vi "practice1-case2-Merve Polat.vi"() -> ()   [LabVIEW 2024]
panel:
  out "Numeric 4":dbl
  out "Ch1 Outflow Tube(4-2)":u32(colorbox)
  out "appended array":i8[](array[numeric]) format="%02x"
  out "Byte 2(8bit integer)":i8
  out "Byte 1(8bit integer)":i8
  out "Numeric 5":dbl
  out "Numeric 3":dbl
  out "Numeric 2":dbl
  out "Numeric":dbl
  out "element":u32
  out "Ch1 Current Digit Color(7-5)":u32(colorbox)
  out "Ch1 Voltage Digit Color(4-2)":u32(colorbox)
  out "Ch1 Frame Color(7-5)":u32(colorbox)
  out "1 o":u32[](array[numeric])
  out "2":u32[](array[numeric])
  out "color":u32[](array[colorbox])
  out "?":string
  out "?":string
  out "?":string
  out "?":string
  in  "Byte Array":u8[](array[numeric]) format="%02x"
  # "Ch1 Current Digit Color"
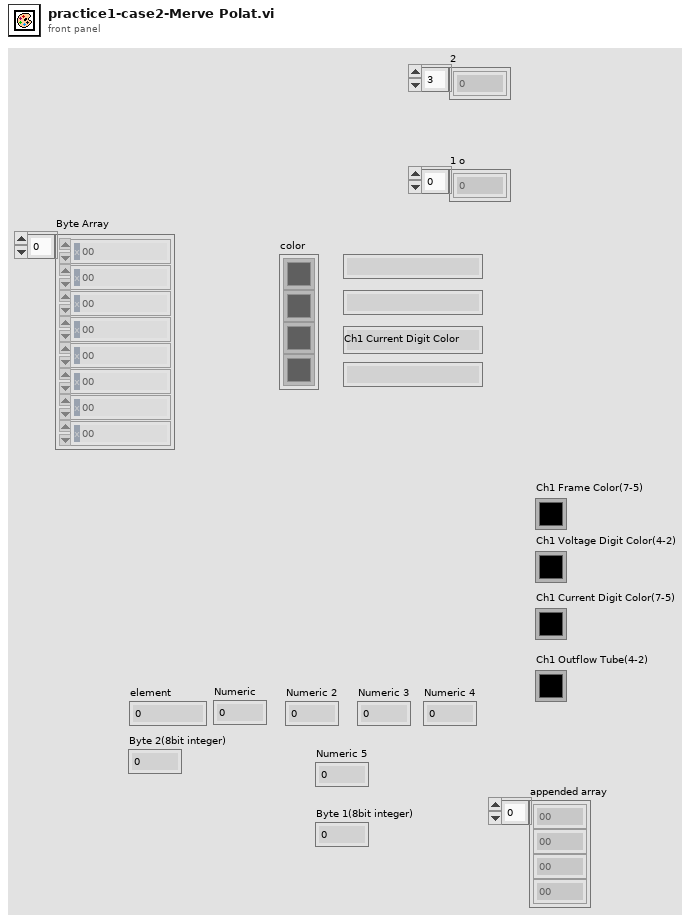
[diagram p1: front panel]
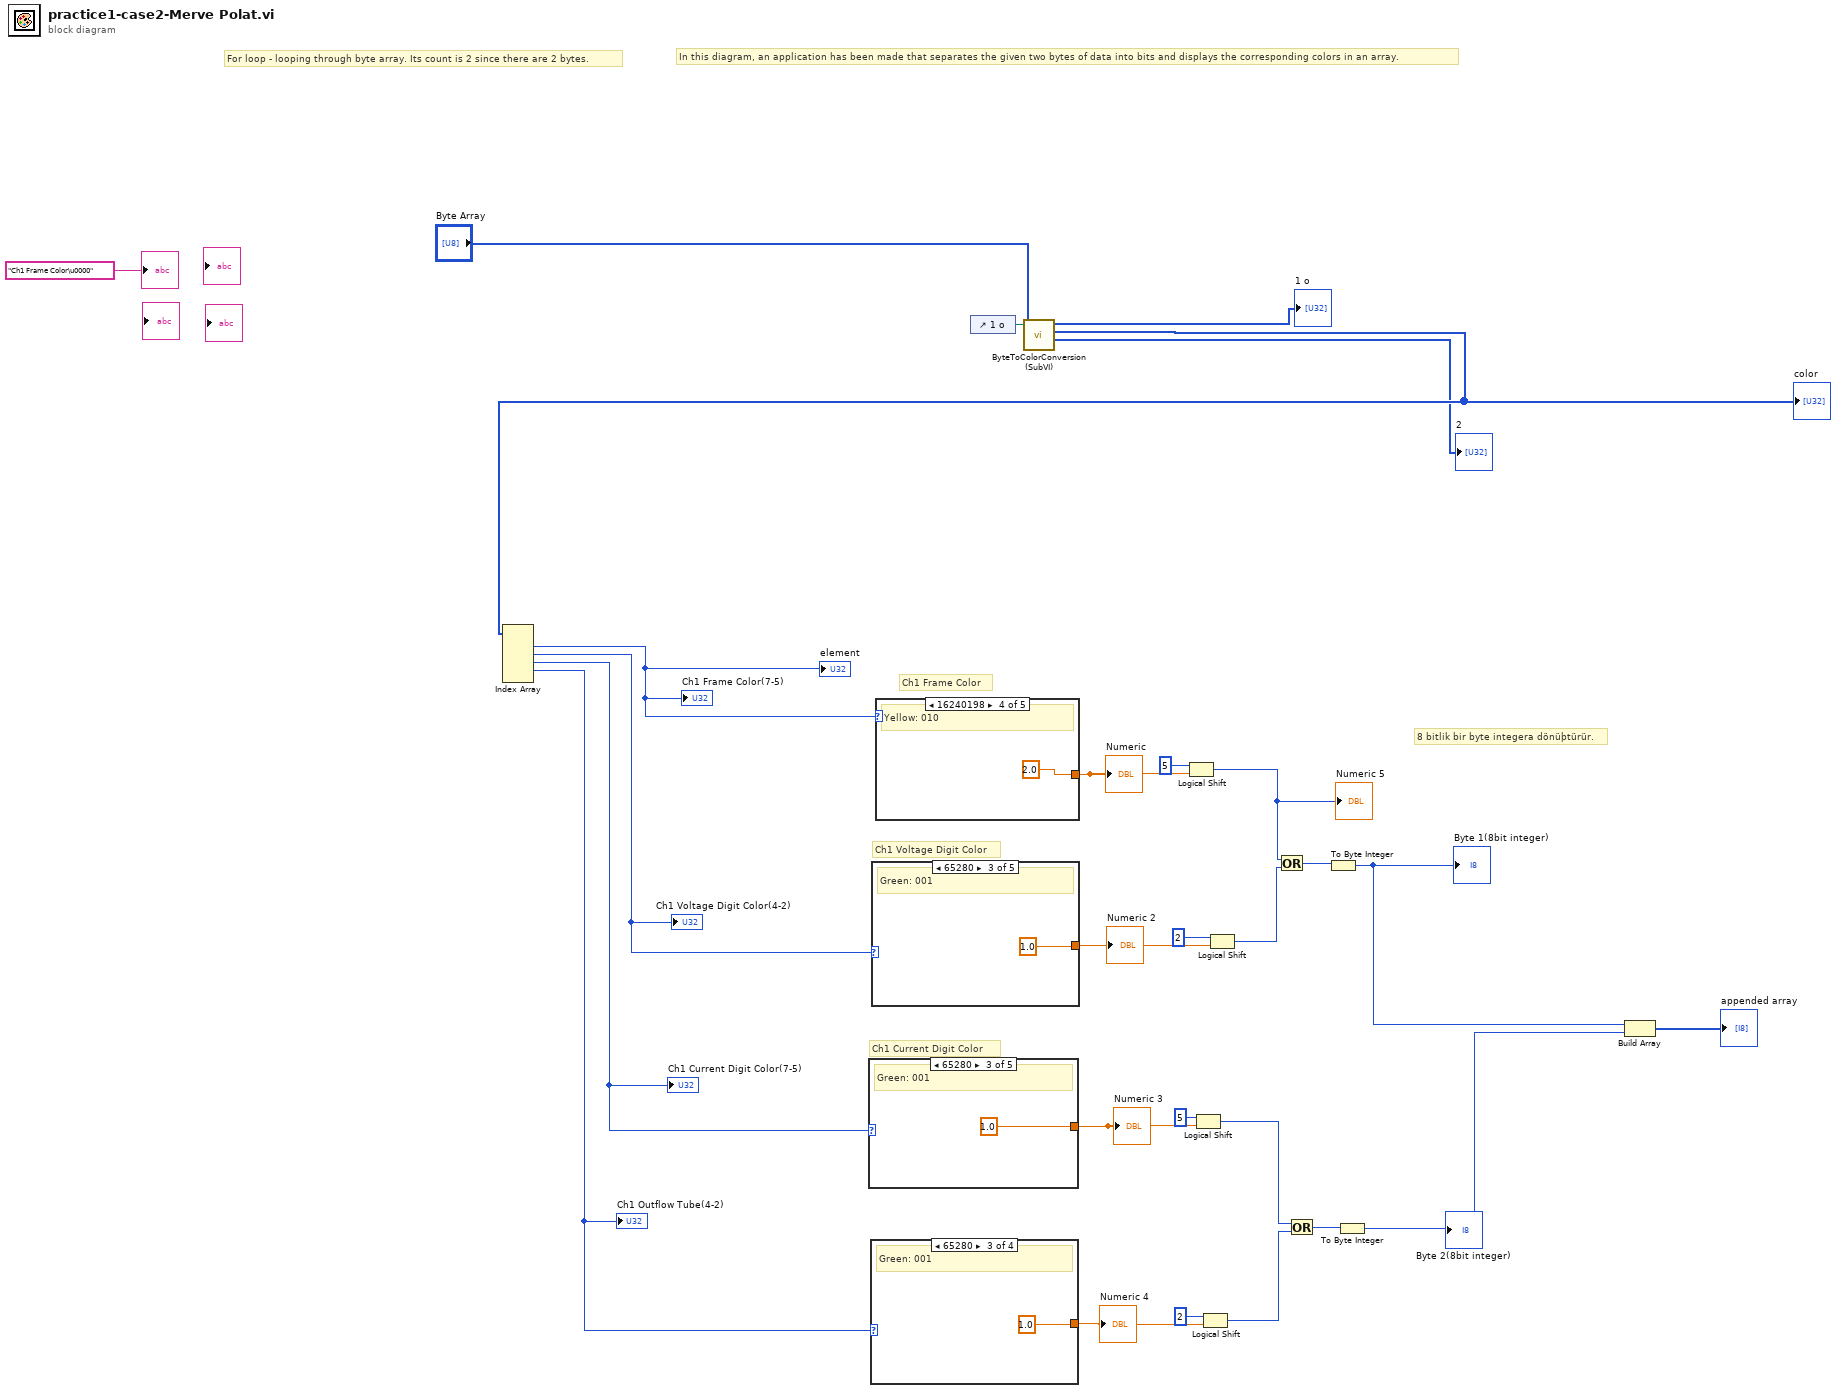
[diagram p0: block diagram]
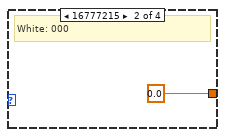
[diagram p3: hidden frame]
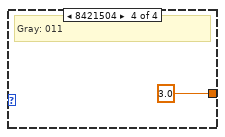
[diagram p4: hidden frame]
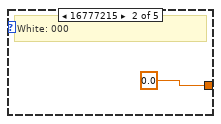
[diagram p6: hidden frame]
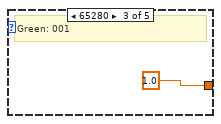
[diagram p7: hidden frame]
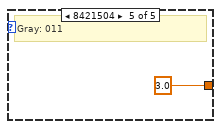
[diagram p8: hidden frame]
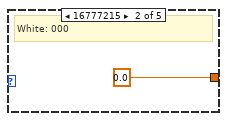
[diagram p10: hidden frame]
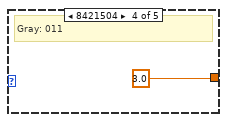
[diagram p11: hidden frame]
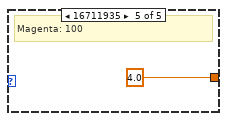
[diagram p12: hidden frame]
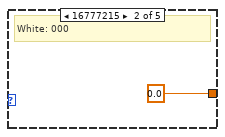
[diagram p14: hidden frame]
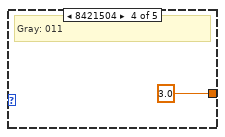
[diagram p15: hidden frame]
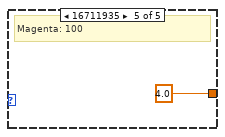
[diagram p16: hidden frame]
diagram:
  # "8 bitlik bir byte integera dönüþtürür."
  # "Ch1 Current Digit Color"
  # "Ch1 Voltage Digit Color"
  # "Ch1 Frame Color"
  # "In this diagram, an application has been made that separates the given two bytes of data into bits and displays the corresponding colors in an array."
  # "For loop - looping through byte array. Its count is 2 since there are 2 bytes."
  n1 = control-ref of="1 o"() -> (w3:refnum<vi>)
  n2 = call "ByteToColorConversion (SubVI).vi"("Byte Array"="Byte Array", "Array in"=w3) -> ("2"=→"2":u32[], "1 o 2"=w13:u32[], "1 o"=→"1 o":u32[])  [unwired: 7 in]
  "color" <- w13
  n3 = Index Array "Index Array"(array=w13) -> (element #1=w26:u32, element #2=w10:u32, element #3=w12:u32, element #4=w9:u32)  [unwired: 5 in, 1 out]
  "Ch1 Frame Color(7-5)" <- w26
  "Ch1 Voltage Digit Color(4-2)" <- w10
  "Ch1 Current Digit Color(7-5)" <- w12
  "element" <- w26
  "Ch1 Outflow Tube(4-2)" <- w9
  n4 = case shown="65280" w12 {
    tunnel: [_ 0.0 ("Numeric 3") 1.0 ("Numeric 3") 3.0 ("Numeric 3") 4.0 ("Numeric 3")] -> w19
    frame Default {
      # "None of these case is true"
    }
    frame 16777215 {
      # "White: 000"
    }
    frame 65280 {
      # "Green: 001"
    }
    frame 8421504 {
      # "Gray: 011"
    }
    frame 16711935 {
      # "Magenta: 100"
    }
  }
  "Numeric 3" <- w19
  n5 = case shown="65280" w9 {
    tunnel: [_ 0.0 ("Numeric") 1.0 ("Numeric") 3.0 ("Numeric")] -> w11
    frame Default {
      # "None of these case is true"
    }
    frame 16777215 {
      # "White: 000"
    }
    frame 65280 {
      # "Green: 001"
    }
    frame 8421504 {
      # "Gray: 011"
    }
  }
  "Numeric 4" <- w11
  n6 = case shown="65280" w10 {
    tunnel: [_ 0.0 ("Numeric") 1.0 ("Numeric") 3.0 ("Numeric") 4.0 ("Numeric")] -> w22
    frame Default {
      # "None of these case is true"
    }
    frame 16777215 {
      # "White: 000"
    }
    frame 65280 {
      # "Green: 001"
    }
    frame 8421504 {
      # "Gray: 011"
    }
    frame 16711935 {
      # "Magenta: 100"
    }
  }
  "Numeric 2" <- w22
  n7 = case shown="16240198" w26 {
    tunnel: [_ 0.0 ("Numeric") 1.0 ("Numeric") 2.0 ("Numeric") 3.0 ("Numeric")] -> w24
    frame Default {
      # "None of these case is true"
    }
    frame 16777215 {
      # "White: 000"
    }
    frame 65280 {
      # "Green: 001"
    }
    frame 16240198 {
      # "Yellow: 010"
    }
    frame 8421504 {
      # "Gray: 011"
    }
  }
  "Numeric" <- w24
  n8 = Logical Shift(y=i16 5, x=w24) -> (x << y=w18:u32)
  "Numeric 5" <- w18
  n9 = Logical Shift(y=i16 5, x=w19) -> (x << y=w7:u32)
  n10 = Logical Shift(y=i16 2, x=w11) -> (x << y=w6:u32)
  n11 = Logical Shift(y=i16 2, x=w22) -> (x << y=w21:u32)
  n12 = Or(x=w18, y=w21) -> (x .or. y?=w17:u32)
  n13 = Or(x=w7, y=w6) -> (x .or. y?=w5:u32)
  n14 = To Byte Integer(number=w17) -> (8bit integer=w16:i8)
  "Byte 1(8bit integer)" <- w16
  n15 = To Byte Integer(number=w5) -> (8bit integer=w15:i8)
  "Byte 2(8bit integer)" <- w15
  n16 = Build Array "Build Array"(w16, w15) -> (→"appended array":i8[])
  "?" <- "Ch1 Frame Color\u0000"
